vi "Go to Position.vi"(9 "Move Straight In":bool, 10 "Goal Frame (World)":cluster{"X":sgl, "Y":sgl, "Theta":dbl}, 11 "Robot Frame (World)":cluster{"X":sgl, "Y":sgl, "Theta":dbl}) -> (1 "Move Straight Out":bool, 2 "Goal Arrive?":bool, 3 "Frame Velocity":dbl[](array[numeric]))   [LabVIEW 2016]
uses:
  <vilib>/Analysis/coordinate.llb/Angle Units.ctl
  <vilib>/Analysis/coordinate.llb/Angle Range (Degree).ctl
  <vilib>/Analysis/coordinate.llb/Wrap Angle (scalar).vi
  <vilib>/Analysis/NI_AAL_Angle.lvlib
panel:
  out "alpha":dbl
  in  "K3 (have to be negative)":dbl=-0.8
  in  "K2":dbl=6.0
  in  "K1":dbl=1.5
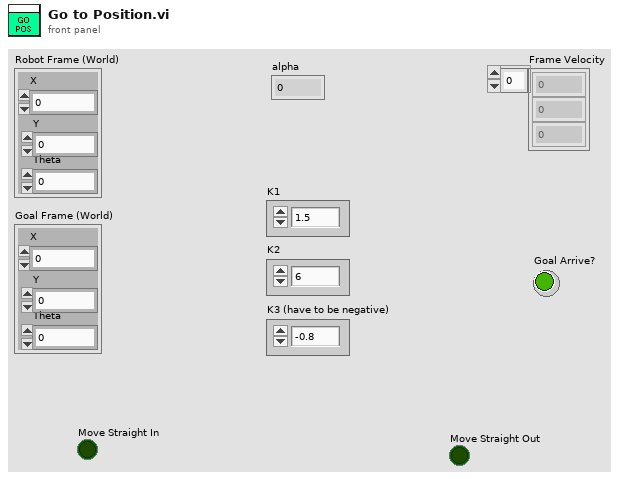
[diagram p1: front panel]
types:
  T1 = typedef "NI_AAL_Angle.lvlib/Angle Range (Degree).ctl" = u16
  T2 = typedef "NI_AAL_Angle.lvlib/Angle Units.ctl" = i32
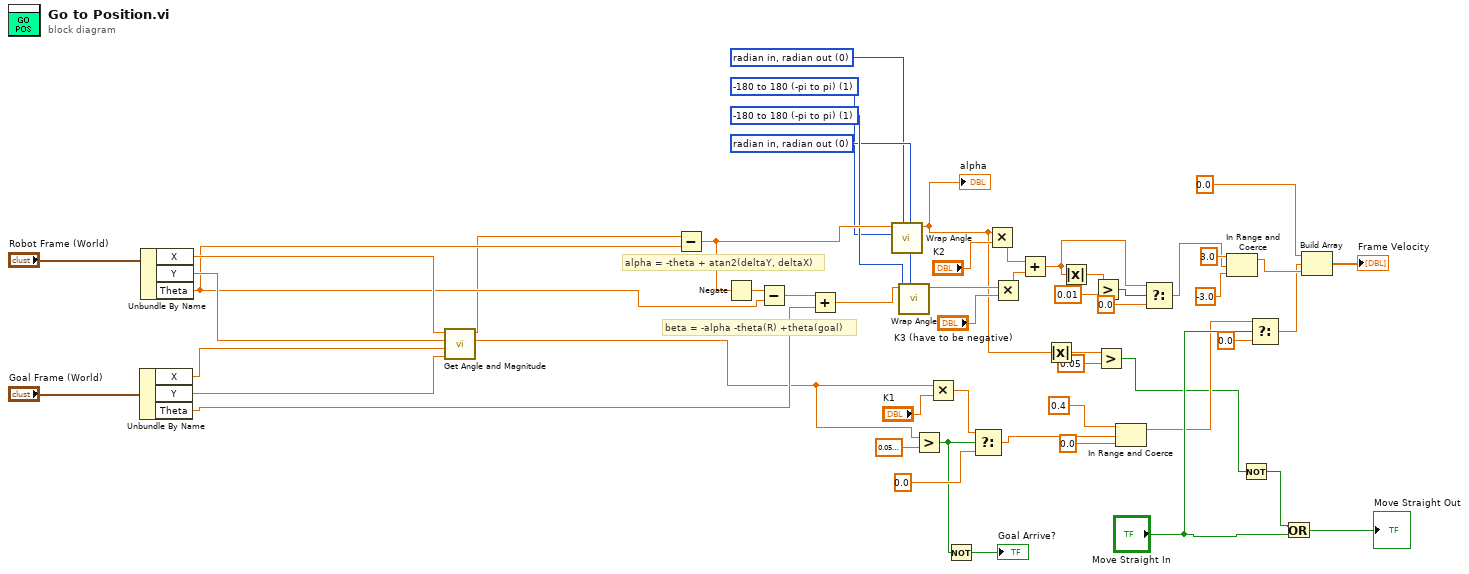
[diagram p0: block diagram]
diagram:
  w43 = T1 1 items=["none", "-180 to 180 (-pi to pi)", "0 to 360 (0 to 2pi)"] ("angle range")
  w44 = T2 0 items=["radian in, radian out", "radian in, degree out", "degree in, degree out", "degree in, radian out"] ("angle units")
  w45 = T2 0 items=["radian in, radian out", "radian in, degree out", "degree in, degree out", "degree in, radian out"] ("angle units")
  w46 = T1 1 items=["none", "-180 to 180 (-pi to pi)", "0 to 360 (0 to 2pi)"] ("angle range")
  # "beta = -alpha -theta(R) +theta(goal)"
  # "alpha = -theta + atan2(deltaY, deltaX)"
  n1 = Unbundle By Name("Goal Frame (World)") -> ("X"=w51:sgl, "Y"=w7:sgl, "Theta"=w22:dbl)
  n2 = Unbundle By Name("Robot Frame (World)") -> ("X"=w50:sgl, "Y"=w49:sgl, "Theta"=w23:dbl)
  n3 = call "Get Angle and Magnitude.vi"("YGoal"=w7, "XGoal"=w51, "Y"=w49, "X"=w50) -> ("Magnitude"=w5:sgl, "Angle Out (rad)"=w6:sgl)  [unwired: 4 in, 2 out]
  n4 = Subtract(x=w6, y=w23) -> (x-y=w47:dbl)
  n5 = Negate(x=w47) -> (-x=w48:dbl)
  n6 = Subtract(x=w48, y=w23) -> (x-y=w21:dbl)
  n7 = Add(x=w21, y=w22) -> (x+y=w20:dbl)
  n8 = call-poly <vilib>:"Wrap Angle.vi"("angle units"=w44, "angle range"=w43, "angle in"=w47) -> ("angle out"=w1:dbl)  [unwired: 7 in, 1 out]
  "alpha" <- w1
  n9 = call-poly <vilib>:"Wrap Angle.vi"("angle units"=w45, "angle range"=w46, "angle in"=w20) -> ("angle out"=w42:dbl)  [unwired: 7 in, 1 out]
  n10 = Greater?(x=w5, y=sgl 0.05) -> (0:w31:bool)
  n11 = Multiply(x=w5, y="K1") -> (x*y=w38:dbl)
  n12 = Not(x=w31) -> (.not. x?=→"Goal Arrive?":bool)
  n13 = Select(t=w38, s=w31, f=sgl 0.0) -> (s? t:f=w29:dbl)
  n14 = Multiply(x=w1, y="K2") -> (x*y=w40:dbl)
  n15 = Multiply(x=w42, y="K3 (have to be negative)") -> (x*y=w41:dbl)
  n16 = Add(x=w40, y=w41) -> (x+y=w18:dbl)
  n17 = Absolute Value(x=w1) -> (abs(x)=w4:dbl)
  n18 = Absolute Value(x=w18) -> (abs(x)=w15:dbl)
  n19 = Greater?(x=w15, y=0.01) -> (0:w13:bool)
  n20 = Greater?(x=w4, y=0.05) -> (0:w2:bool)
  n21 = In Range and Coerce(upper limit=0.4, x=w29, lower limit=0.0) -> (coerced(x)=w10:dbl)  [unwired: 1 out]
  n22 = Select(t=w18, s=w13, f=0.0) -> (s? t:f=w16:dbl)
  n23 = In Range and Coerce(upper limit=3.0, x=w16, lower limit=-3.0) -> (coerced(x)=w24:dbl)  [unwired: 1 out]
  n24 = Not(x=w2) -> (.not. x?=w12:bool)
  n25 = Select(t=w10, s="Move Straight In", f=0.0) -> (s? t:f=w8:dbl)
  n26 = Or(x=w12, y="Move Straight In") -> (x .or. y?=→"Move Straight Out":bool)
  n27 = Build Array(0.0 ("index"), w8, w24) -> (→"Frame Velocity":dbl[])
